vi "Initialize Routing and Faulting Custom Device.vi"(8 "error in":errorcluster, 11 "routing and faulting custom device in":T1 format="%.0x") -> (0 "error out":errorcluster, 1 "routing channels":T1 format="%.0x", 2 "endpoint aliases":T1 format="%.0x", 3 "routing and faulting custom device out":T1 format="%.0x")   [LabVIEW 2020, in "Routing and Faulting Scripting.lvlib"]
uses:
  Routing and Faulting Scripting.lvlib
  <vilib>/NI VeriStand/Custom Device API/Custom Device Item Ref.ctl
  Shared/Constants.vi
  <vilib>/NI VeriStand/Custom Device API/Custom Device API.lvlib
  Dependencies.llb/Routing and Faulting Shared.lvlib
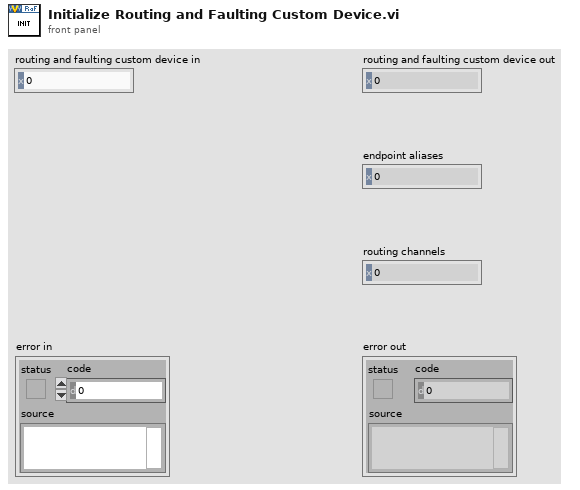
[diagram p1: front panel]
types:
  T1 = typedef "Custom Device API.lvlib/Custom Device Item Ref.ctl" = u64
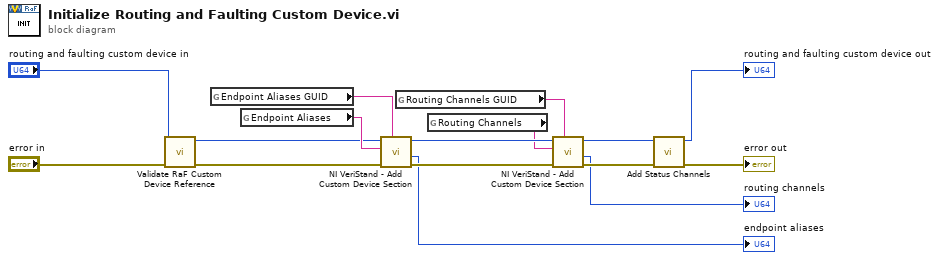
[diagram p0: block diagram]
diagram:
  n1 = call "Validate RaF Custom Device Reference.vi"("error in"="error in", "routing and faulting in"="routing and faulting custom device in") -> ("error out"=w3:errorcluster, "routing and faulting out"=w1:T1)  [unwired: 8 in]
  n2 = global read "Constants.vi" "Endpoint Aliases GUID"() -> (w11:string)
  n3 = global read "Constants.vi" "Endpoint Aliases"() -> (w13:string)
  n4 = call <vilib>:"NI VeriStand - Add Custom Device Section.vi"("GUID (Default Section)"=w11, "error in (no error)"=w3, "Section Name"=w13, "Parent Ref in"=w1) -> ("error out"=w15:errorcluster, "Section Ptr"=→"endpoint aliases":T1, "Parent Ref out"=w16:T1)  [unwired: 4 in, 1 out]
  n5 = global read "Constants.vi" "Routing Channels GUID"() -> (w10:string)
  n6 = global read "Constants.vi" "Routing Channels"() -> (w12:string)
  n7 = call <vilib>:"NI VeriStand - Add Custom Device Section.vi"("GUID (Default Section)"=w10, "error in (no error)"=w15, "Section Name"=w12, "Parent Ref in"=w16) -> ("error out"=w14:errorcluster, "Section Ptr"=→"routing channels":T1, "Parent Ref out"=w6:T1)  [unwired: 4 in, 1 out]
  n8 = call "Add Status Channels.vi"("error in"=w14, "routing and faulting custom device in"=w6) -> ("error out"=→"error out":errorcluster, "routing and faulting custom device out"=→"routing and faulting custom device out":T1)  [unwired: 8 in]
